vi "PIDtest.vi"() -> ()   [LabVIEW 2015]
uses:
  <vilib>/addons/control/pid/pid.llb/PID (DBL).vi
  <vilib>/addons/control/pid/NI_PID_pid.lvlib
panel:
  in  "stop":bool
  in  "PID gains":T1={"proportional gain (Kc)"=1.0, "integral time (Ti, min)"=0.01, "derivative time (Td, min)"=0.0} {"derivative time (Td, min)" format="%.3f"; "integral time (Ti, min)" format="%.3f"; "proportional gain (Kc)" format="%.3f"}
  in  "Slide":dbl(slide) scale=0.0..10.0
  out "Meter":dbl(knob) scale=0.0..10.0
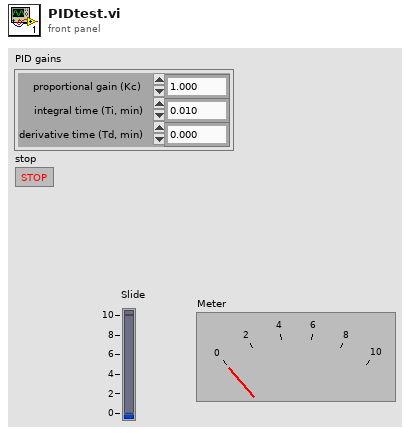
[diagram p1: front panel]
types:
  T1 = cluster{"proportional gain (Kc)":dbl, "integral time (Ti, min)":dbl, "derivative time (Td, min)":dbl}
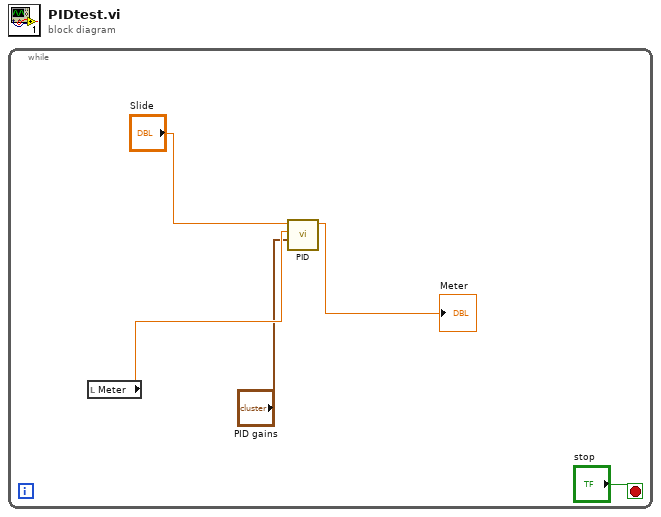
[diagram p0: block diagram]
diagram:
  n1 = while {
    stop <- "stop" stop-if-true
    n2 = local read "Meter"() -> (w5:dbl)
    n3 = call-poly <vilib>:"PID.vi"("PID gains"="PID gains", "process variable"=w5, "setpoint"="Slide") -> ("output"=→"Meter":dbl)  [unwired: 7 in, 1 out]
  }
